vi "Tencion Conversion.vi"(8 "error in":errorcluster, 10 "Enum":T1, 11 "Tencion Input":dbl) -> (0 "error out":errorcluster, 3 "Tencion [kgf]":dbl)   [LabVIEW 2025]
uses:
  Controls/Tencion Conversion Table.ctl
  Controls/Spork type.ctl
panel:
  out "Array":dbl[](array[numeric])
  in  "Tencion Conversion Table":T2
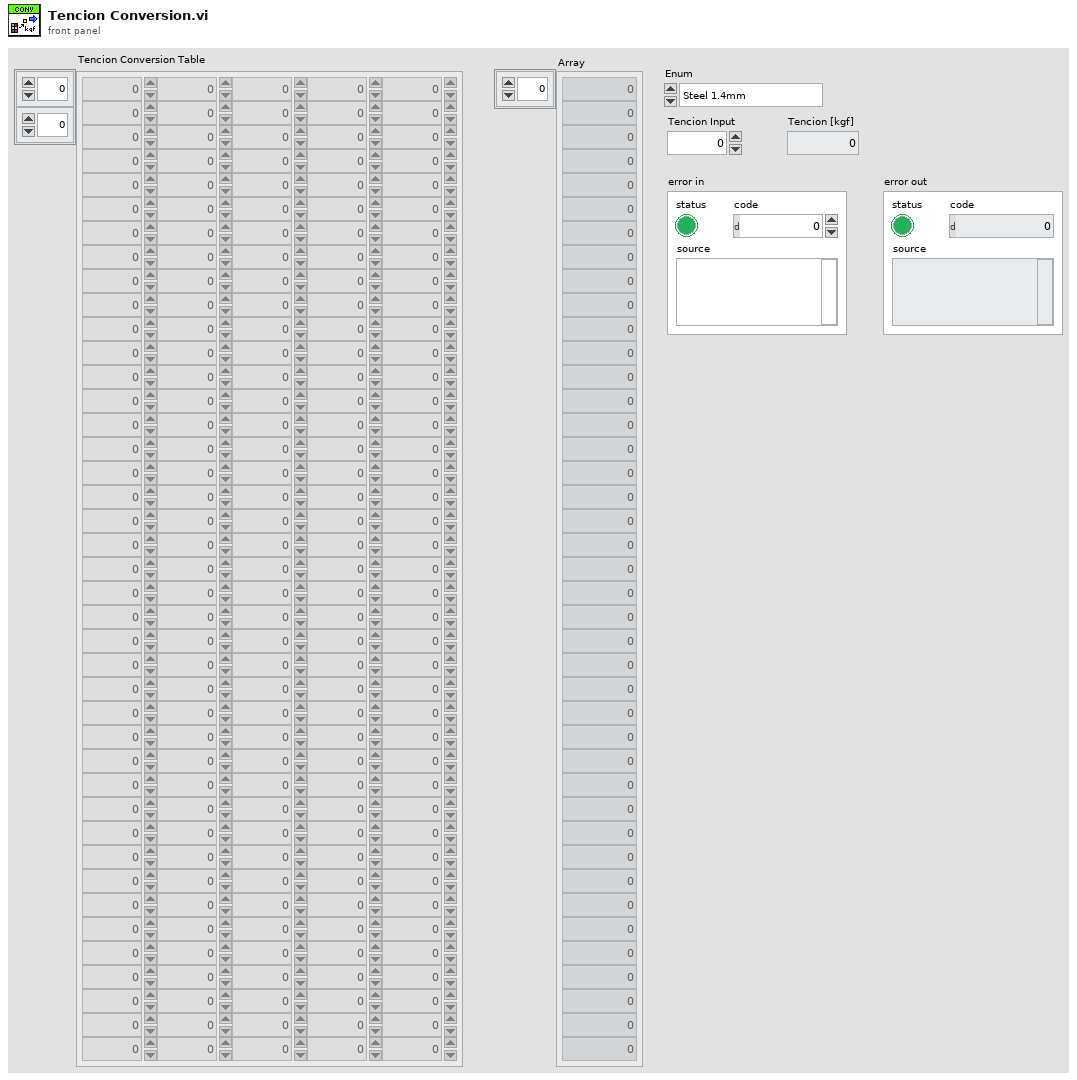
[diagram p1: front panel]
types:
  T1 = typedef "Spork type.ctl" = enum16{"Steel 1.4mm", "Steel 1.5mm", "Steel 1.6mm", "Steel 1.7mm", "Steel 1.8mm", "Steel 2mm", "Steel 2.3mm", "Steel 2.5mm", "Steel 2.6mm", "Aluminum 2.28mm", "Aluminum 2.54mm", "Aluminum 2.8mm", "Aluminum 3.3mm"}
  T2 = typedef "Tencion Conversion Table.ctl" = dbl[][]
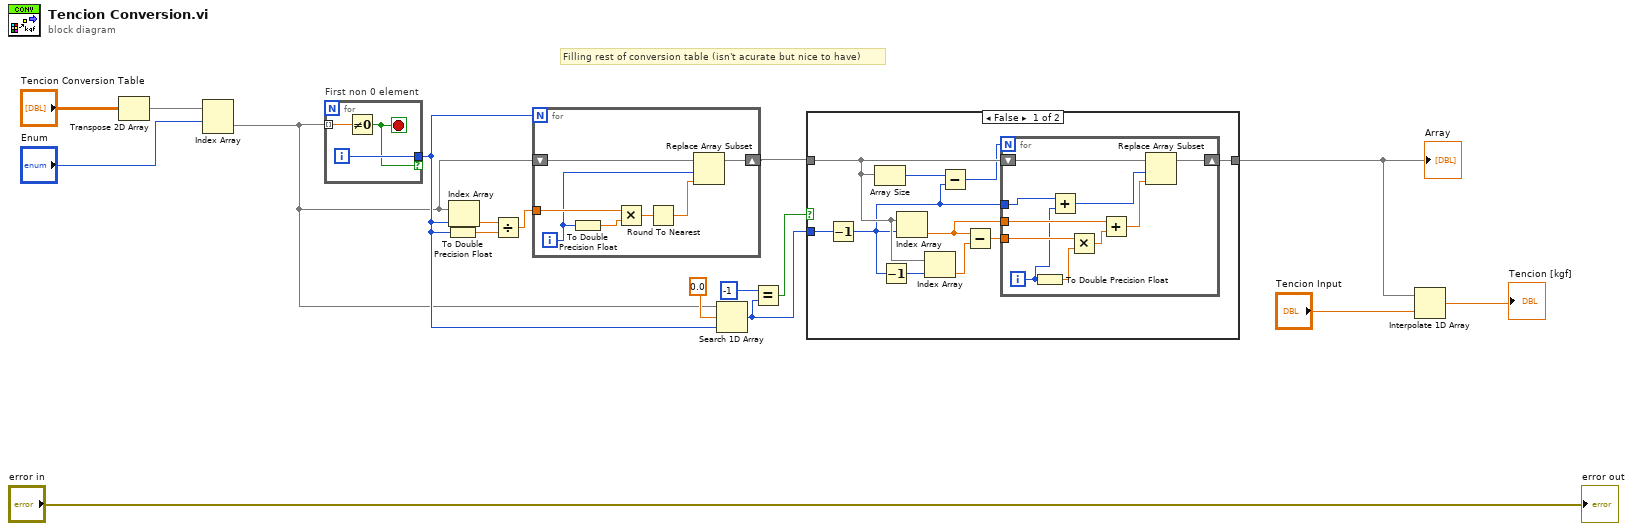
[diagram p0: block diagram]
diagram:
  # "Filling rest of conversion table (isn't acurate but nice to have)"
  n1 = Transpose 2D Array(2D array="Tencion Conversion Table") -> (transposed array=w6:T2)
  n2 = Index Array(array=w6, index (row)="Enum") -> (element=w7:dbl[])  [unwired: 1 in]
  n3 = for "First non 0 element" {
    tunnel: w7 -> [w20] mode=indexing
    tunnel: [w19] -> w13 if=w18
    i -> [w19]
    stop <- w18 stop-if-true
    n4 = Not Equal To 0?(x=w20) -> (x != 0?=w18:bool)
  }
  n5 = To Double Precision Float(number=w13) -> (double precision float=w15:dbl)
  n6 = Index Array(array=w7, index=w13) -> (element=w16:dbl)
  n7 = Divide(x=w16, y=w15) -> (x/y=w14:dbl)
  n8 = for {
    N: w13 -> [_]
    tunnel: w14 -> [w26]
    shift-right: [w23] -> w11
    shift-left: w7 -> [w27]
    i -> [w24]
    n9 = To Double Precision Float(number=w24) -> (double precision float=w25:dbl)
    n10 = Multiply(x=w26, y=w25) -> (x*y=w22:dbl)
    n11 = Round To Nearest(number=w22) -> (nearest integer value=w21:dbl)
    n12 = Replace Array Subset(array=w27, new element=w21, index=w24) -> (w23:dbl[])
  }
  n13 = Search 1D Array(1D array=w7, element=0.0, start index (0)=w13) -> (index of element=w8:i32)
  n14 = Equal?(x=-1, y=w8) -> (x = y?=w9:bool)
  n15 = case shown="False" w9 {
    tunnel: [w31 w48] -> w2
    tunnel: w11 -> [w33 w48]
    tunnel: w8 -> [w30 _]
    frame False {
      n16 = Decrement(x=w30) -> (x-1=w28:i32)
      n17 = Array Size(array=w33) -> (size(s)=w35:i32)
      n18 = Decrement(x=w28) -> (x-1=w37:i32)
      n19 = Index Array(array=w33, index=w28) -> (element=w32:dbl)
      n20 = Index Array(array=w33, index=w37) -> (element=w36:dbl)
      n21 = Subtract(x=w35, y=w28) -> (x-y=w29:i32)
      n22 = Subtract(x=w32, y=w36) -> (x-y=w34:dbl)
      n23 = for {
        N: w29 -> [_]
        tunnel: w34 -> [w46]
        tunnel: w32 -> [w43]
        shift-right: [w41] -> w31
        shift-left: w33 -> [w47]
        tunnel: w28 -> [w38]
        i -> [w40]
        n24 = To Double Precision Float(number=w40) -> (double precision float=w45:dbl)
        n25 = Add(x=w38, y=w40) -> (x+y=w39:i32)
        n26 = Multiply(x=w46, y=w45) -> (x*y=w44:dbl)
        n27 = Add(x=w43, y=w44) -> (x+y=w42:dbl)
        n28 = Replace Array Subset(array=w47, new element=w42, index=w39) -> (w41:dbl[])
      }
    }
    frame True {
    }
  }
  "Array" <- w2
  n29 = Interpolate 1D Array(1:"Tencion Input", 2:w2) -> (0:→"Tencion [kgf]":dbl)
  "error out" <- "error in"
